vi "tcsOfc_getNextSample_loopTimeMs.vi"(8 "error in (no error)":errorcluster, 11 "loopTimeMs_Ctl":T1) -> (0 "error out":errorcluster, 2 "function return":i32, 3 "loopTimeMs_Ctl out":T1)   [LabVIEW 2016, in "SALLV_tcsOfc.lvlib"]
doc: "int tcsOfc_shm_getNextSample_loopTimeMsLV(tcsOfc_loopTimeMsLV *loopTimeMs_Ctl );"
uses:
  SALLV_tcsOfc.lvlib
  DataTypes/loopTimeMs.ctl
  SALLV_tcsOfc.so
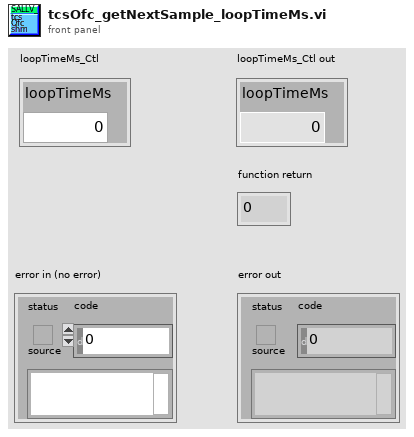
[diagram p1: front panel]
types:
  T1 = typedef "SALLV_tcsOfc.lvlib/loopTimeMs.ctl" = cluster{"loopTimeMs":dbl}
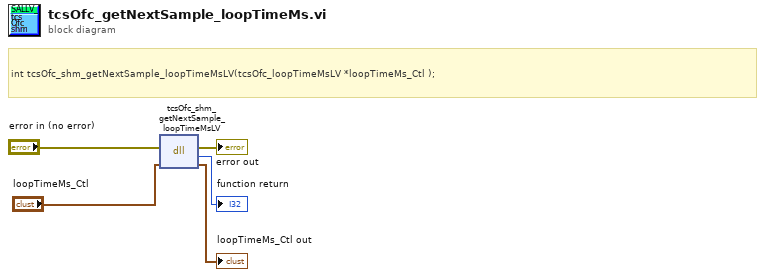
[diagram p0: block diagram]
diagram:
  # "int tcsOfc_shm_getNextSample_loopTimeMsLV(tcsOfc_loopTimeMsLV *loopTimeMs_Ctl );"
  n1 = dll-call lib="home/ttsai/Documents/salAPI/SALLV_tcsOfc.*" fn="tcsOfc_shm_getNextSample_loopTimeMsLV"(error in="error in (no error)", "loopTimeMs_Ctl"="loopTimeMs_Ctl") -> (error out=→"error out":errorcluster, →"function return":i32, "loopTimeMs_Ctl"=→"loopTimeMs_Ctl out":T1)  [unwired: 2 in, 1 out]
